vi "Write JUnit Report.vi"(9 "Project Name":string, 10 "Test Results":refnum<class "Test Result.lvclass">[](array[class]), 11 "File Path":path) -> (0 "error out":errorcluster)   [LabVIEW 2017, in "JUnit.lvlib"]
uses:
  JUnit.lvlib
  Test Result/Test Result.lvclass
  Test Result/Test Result.lvclass/Test Result.ctl
  Test Case/Test Case.lvclass/Test Case.ctl
  Test Result/Get Start Time.vi
  Test Result/Get Outcome.vi
  Test Result/Get Failure Message.vi
  Test Result/Get End Time.vi
  Test Result/Get Test Case.vi
  Test Case/Get Qualified Name.vi
  <vilib>/PNR/JUnit XML/JUnit XML/Test Suite/Write Timestamp.vi
  Test Case/Test Case.lvclass
  <vilib>/PNR/JUnit XML/JUnit XML/Test Suite/Test Suite.lvclass
  <vilib>/PNR/JUnit XML/JUnit XML/Test Case/Test Case.lvclass
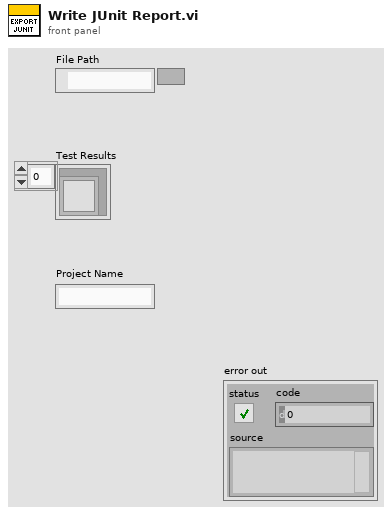
[diagram p1: front panel]
types:
  T1 = typedef "Test Outcome.ctl" = enum16{"None", "Passed", "Failed"}
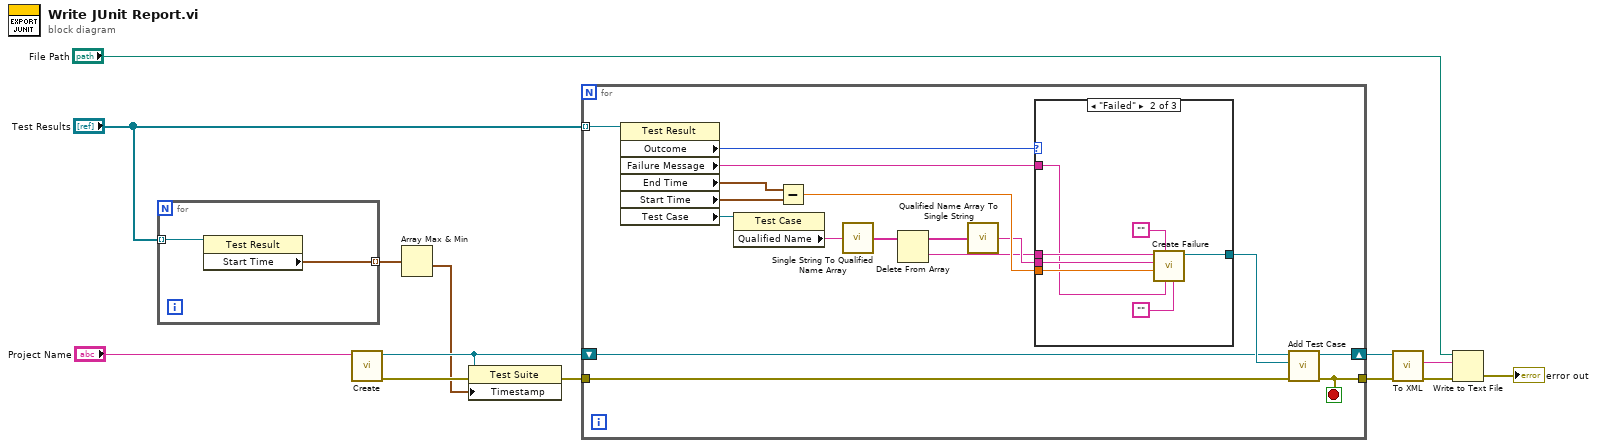
[diagram p0: block diagram]
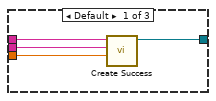
[diagram p2: hidden frame]
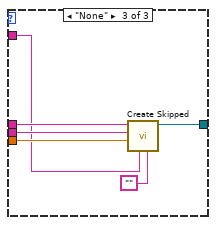
[diagram p3: hidden frame]
diagram:
  n1 = for {
    tunnel: "Test Results" -> [w15] mode=indexing
    tunnel: [w14] -> w12 mode=indexing
    n2 = property class="Test Result"(reference=w15) -> ("Start Time"=w14:timestamp)  [unwired: 1 in, 2 out]
  }
  n3 = call <vilib>:"Create.vi"("Name"="Project Name") -> ("error out"=w9:errorcluster, "Test Suite"=w6:refnum<class "Test Suite.lvclass">)  [unwired: 9 in]
  n4 = Array Max & Min(array=w12) -> (min value=w5:timestamp)  [unwired: 3 out]
  n5 = property class="Test Suite"(reference=w6, error in=w9, "Timestamp"=w5) -> (error out=w7:errorcluster)  [unwired: 1 out]
  n6 = for {
    tunnel: "Test Results" -> [w32] mode=indexing
    shift-right: [w18] -> w2
    shift-left: w6 -> [w19]
    tunnel: w7 -> [w17]
    tunnel: [w16] -> w1
    stop <- w16 stop-if-true
    n7 = property class="Test Result"(reference=w32) -> ("Outcome"=w30:T1, "Failure Message"=w29:string, "End Time"=w27:timestamp, "Start Time"=w28:timestamp, "Test Case"=w31:refnum<class "Test Case.lvclass">)  [unwired: 1 in, 2 out]
    n8 = property class="Test Case"(reference=w31) -> ("Qualified Name"=w26:string)  [unwired: 1 in, 2 out]
    n9 = Subtract(x=w27, y=w28) -> (x-y=w23:dbl)
    n10 = call <vilib>:"Single String To Qualified Name Array.vi"("Fully Qualified String"=w26) -> ("Fully Qualified Array"=w25:string[])
    n11 = Delete From Array(array=w25) -> (deleted portion=w21:string, array with subset deleted=w24:string[])  [unwired: 2 in]
    n12 = call <vilib>:"Qualified Name Array To Single String.vi"("Fully Qualified Array"=w24) -> ("Fully Qualified String"=w22:string)
    n13 = case shown="\"Failed\"" w30 {
      tunnel: w29 -> [_ w39 w46]
      tunnel: w23 -> [w36 w41 w47]
      tunnel: w22 -> [w35 w42 w48]
      tunnel: w21 -> [w34 w43 w49]
      tunnel: [w33 w38 w44] -> w20
      frame Default {
        n14 = call <vilib>:"Create Success.vi"("Time"=w36, "Classname"=w35, "Name"=w34) -> ("Test Case"=w33:refnum<class "Test Case.lvclass">)  [unwired: 7 in, 1 out]
      }
      frame "Failed" {
        n15 = call <vilib>:"Create Failure.vi"("Stack Trace"="", "Message"=w39, "Type"="", "Time"=w41, "Classname"=w42, "Name"=w43) -> ("Test Case"=w38:refnum<class "Test Case.lvclass">)  [unwired: 4 in, 1 out]
      }
      frame "None" {
        n16 = call <vilib>:"Create Skipped.vi"("Stack Trace"="", "Message"=w46, "Time"=w47, "Classname"=w48, "Name"=w49) -> ("Test Case"=w44:refnum<class "Test Case.lvclass">)  [unwired: 5 in, 1 out]
      }
    }
    n17 = call <vilib>:"Add Test Case.vi"("error in (no error)"=w17, "Test Case"=w20, "Test Suite in"=w19) -> ("error out"=w16:errorcluster, "Test Suite out"=w18:refnum<class "Test Suite.lvclass">)  [unwired: 7 in]
  }
  n18 = call-dynamic "To XML.vi"("error in (no error)"=w1, "Serializable in"=w2) -> ("error out"=w11:errorcluster, "XML"=w3:string)  [unwired: 8 in]
  n19 = Write to Text File(file (use dialog)="File Path", text=w3, error in=w11) -> (error out=→"error out":errorcluster)  [unwired: 1 in, 2 out]
